vi "HAB Climber.vi"() -> ()   [LabVIEW 2018]
uses:
  <vilib>/Rock Robotics/SystemInterfaces/DIO/FPGA_DIOChannel.ctl
  <vilib>/Rock Robotics/WPI/ThirdParty/Phoenix-LabVIEW/Motor Controller/Controls/CTRE_Phoenix_MotorControl_ControlMode.ctl
  HAB Climber Global.vi
  <vilib>/Rock Robotics/WPI/Switch/WPI_SwitchOpenLimit.vi
  Times/Times Global.vi
  Controllers/Driver Controller/Driver Controller Global.vi
  Cargo Intake/Cargo Intake Global.vi
panel:
  out "HAB Lock":bool
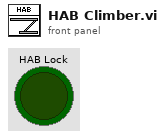
[diagram p1: front panel]
types:
  T1 = typedef "FPGA_DIOChannel.ctl" = enum8{"DIO 0", "DIO 1", "DIO 2", "DIO 3", "DIO 4", "DIO 5", "DIO 6", "DIO 7", "DIO 8", "DIO 9", "DIO MXP 0", "DIO MXP 1", "DIO MXP 2", "DIO MXP 3", "DIO MXP 4", "DIO MXP 5", "DIO MXP 6", "DIO MXP 7", "DIO MXP 8", "DIO MXP 9", "DIO MXP 10", "DIO MXP 11", "DIO MXP 12", "DIO MXP 13", "DIO MXP 14", "DIO MXP 15", "SPI Port CS1", "SPI Port CS2", "SPI Port CS3", "SPI Port MISO", "SPI Port MOSI", "Invalid"}
  T2 = enum16{"HAB Climber Full Manual Mode", "HAB Climber Manual Mode", "HAB Climber Automated Mode", "HAB Climber Fully Automated Mode"}
  T3 = typedef "WPI_SwitchDevRef.ctl" = cluster{"DevStatus":errorcluster, "DIO Channel":T1, "CntIndex":T4, "Normally Closed":bool}
  T4 = typedef "FPGA_CounterCtrSystemIndex.ctl" = enum8{"Ctr 0", "Ctr 1", "Ctr 2", "Ctr 3", "Ctr 4", "Ctr 5", "Ctr 6", "Ctr 7", "Invalid"}
  T5 = typedef "WPI_MotorControlDeviceRef.ctl" = cluster{"DeviceStatus":errorcluster, "Type":T6, "PWM":cluster{"PWM Channel":T7, "DeadBand":T8}, "CAN":cluster{"Device Number":u8, "SetOutput VI Ref":variant, "GetOutput VI Ref":variant, "Enable VI Ref":variant, "Disable VI Ref":variant, "Data":variant}, "Invert":bool, "DIO PWM":cluster{"PWM \"Enable\" Channel":T7, "DIOChannel":T1, "PWM Rate":dbl}}
  T6 = typedef "WPI_MotorControlType.ctl" = enum16{"PWM", "CAN", "DIO PWM"}
  T7 = typedef "FPGA_DIOPWMChannel.ctl" = enum8{"PWM 0", "PWM 1", "PWM 2", "PWM 3", "PWM 4", "PWM 5", "PWM 6", "PWM 7", "PWM 8", "PWM 9", "PWM MXP 0", "PWM MXP 1", "PWM MXP 2", "PWM MXP 3", "PWM MXP 4", "PWM MXP 5", "PWM MXP 6", "PWM MXP 7", "PWM MXP 8", "PWM MXP 9", "Invalid"}
  T8 = typedef "WPI_PWMDeadband.ctl" = cluster{"Name":string, "maxPositivePwm":i32, "minPositivePwm":i32, "centerPwm":i32, "maxNegativePwm":i32, "minNegativePwm":i32, "angularRange":u16}
  T9 = typedef "Control 3.ctl" = dbl
  T10 = typedef "CTRE_Phoenix_MotorControl_ControlMode.ctl" = u16
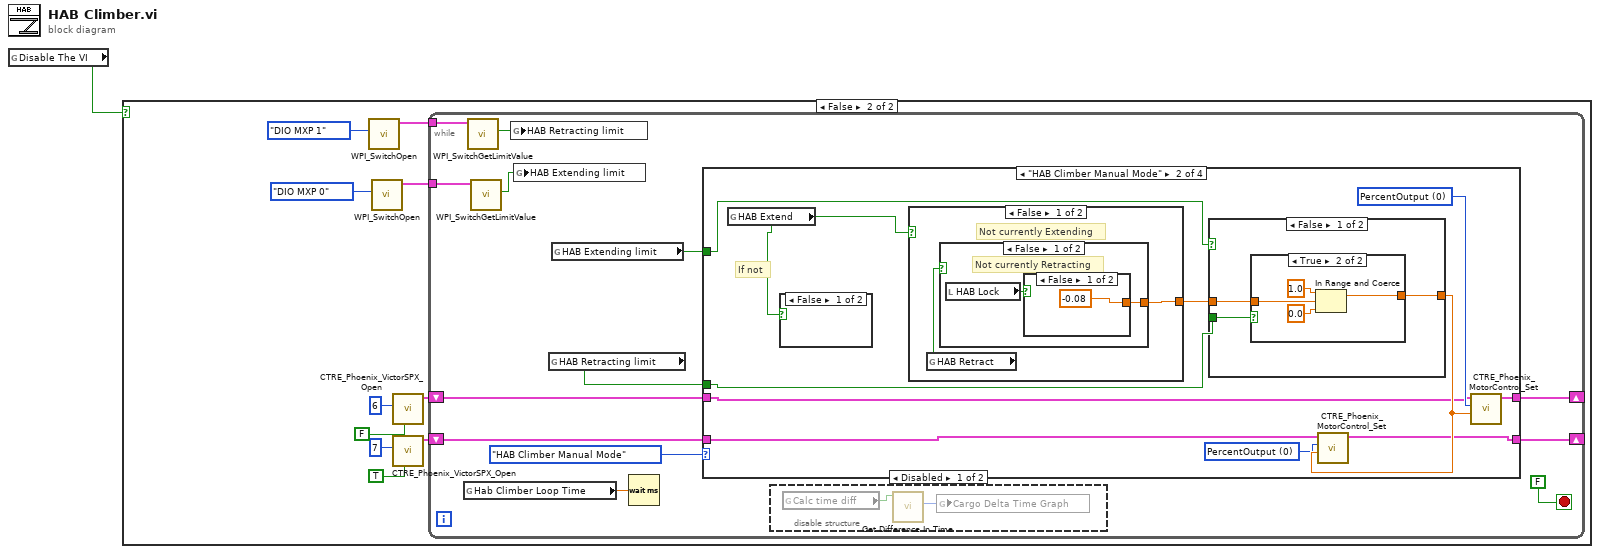
[diagram p0: block diagram]
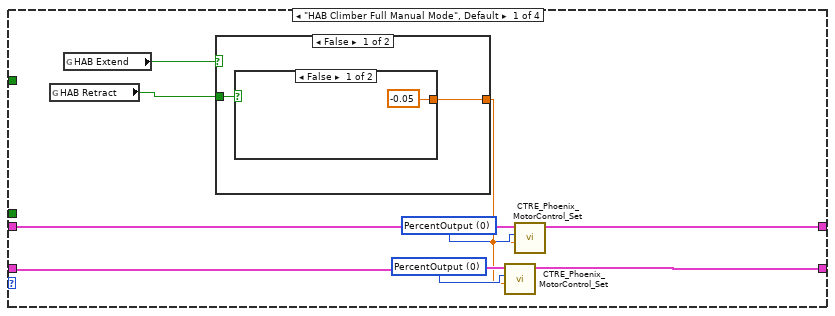
[diagram p4: hidden frame]
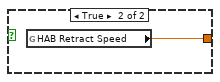
[diagram p5: hidden frame]
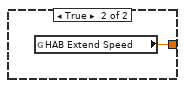
[diagram p6: hidden frame]
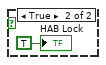
[diagram p7: hidden frame]
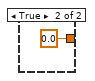
[diagram p8: hidden frame]
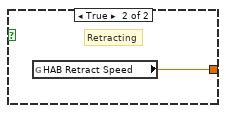
[diagram p9: hidden frame]
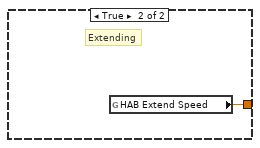
[diagram p10: hidden frame]
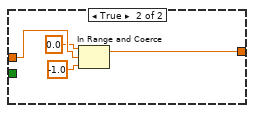
[diagram p12: hidden frame]
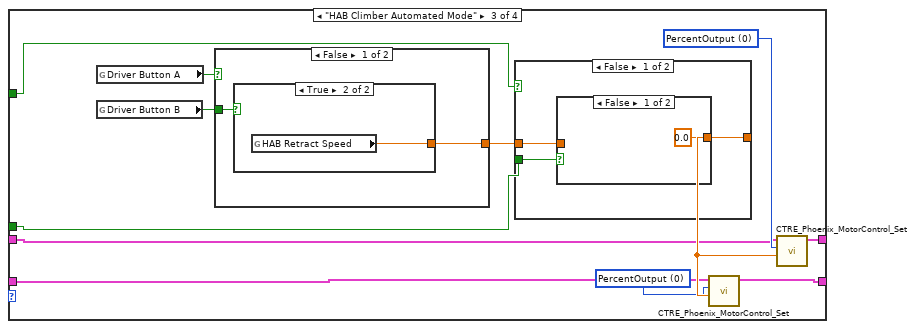
[diagram p13: hidden frame]
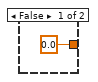
[diagram p14: hidden frame]
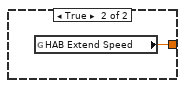
[diagram p15: hidden frame]
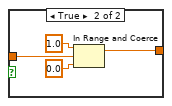
[diagram p16: hidden frame]
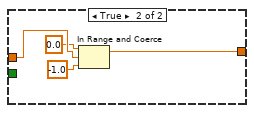
[diagram p17: hidden frame]
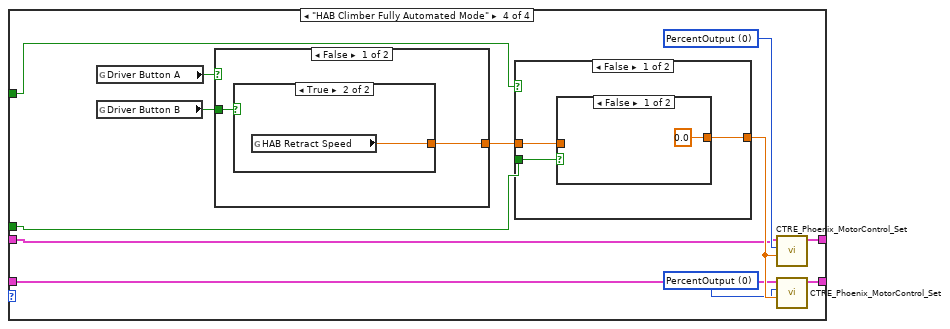
[diagram p18: hidden frame]
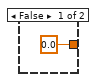
[diagram p19: hidden frame]
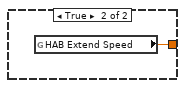
[diagram p20: hidden frame]
diagram:
  n1 = global read "HAB Climber Global.vi" "Disable The VI"() -> (w1:bool)
  n2 = case shown="False" w1 {
    frame True {
    }
    frame False {
      n3 = call-poly <vilib>:"WPI_SwitchOpen.vi"("DIO Channel"=FPGA_DIOChannel."DIO MXP 1") -> ("SwitchDevRef"=w5:T3)  [unwired: 9 in, 1 out]
      n4 = call-poly <vilib>:"WPI_SwitchOpen.vi"("DIO Channel"=FPGA_DIOChannel."DIO MXP 0") -> ("SwitchDevRef"=w4:T3)  [unwired: 9 in, 1 out]
      n5 = call <vilib>:"CTRE_Phoenix_VictorSPX_Open.vi"("Invert"=FALSE, "Device Number"=u8 6) -> ("CAN Talon SRX Ref"=w11:T5)  [unwired: 8 in, 1 out]
      n6 = call <vilib>:"CTRE_Phoenix_VictorSPX_Open.vi"("Invert"=TRUE, "Device Number"=u8 7) -> ("CAN Talon SRX Ref"=w9:T5)  [unwired: 8 in, 1 out]
      n7 = while {
        shift-right: [w19] -> _
        shift-left: w11 -> [w21]
        shift-right: [w18] -> _
        shift-left: w9 -> [w20]
        tunnel: w5 -> [w17]
        tunnel: w4 -> [w16]
        stop <- FALSE stop-if-true
        n8 = global read "Times Global.vi" "Hab Climber Loop Time"() -> (w24:T9)
        n9 = call <vilib>:"WPI_SwitchGetLimitValue.vi"("SwitchDevRef"=w17) -> ("Switch Pressed"=w12:bool)  [unwired: 8 in, 2 out]
        n10 = call <vilib>:"WPI_SwitchGetLimitValue.vi"("SwitchDevRef"=w16) -> ("Switch Pressed"=w13:bool)  [unwired: 8 in, 2 out]
        n11 = global write "HAB Climber Global.vi" "HAB Retracting limit"(w12) -> ()
        n12 = global write "HAB Climber Global.vi" "HAB Extending limit"(w13) -> ()
        n13 = global read "HAB Climber Global.vi" "HAB Retracting limit"() -> (w14:bool)
        n14 = global read "HAB Climber Global.vi" "HAB Extending limit"() -> (w15:bool)
        n15 = Wait (ms)(milliseconds to wait=w24) -> ()  [unwired: 1 out]
        n16 = case shown="\"HAB Climber Manual Mode\"" T2."HAB Climber Manual Mode" ("Mode") {
          tunnel: w21 -> [w32 w47 w78 w107]
          tunnel: w20 -> [w33 w46 w77 w106]
          tunnel: [w30 w45 w76 w105] -> w19
          tunnel: [w29 w44 w75 w104] -> w18
          tunnel: w15 -> [_ w43 w74 w103]
          tunnel: w14 -> [_ w42 w73 w102]
          frame "HAB Climber Full Manual Mode", Default {
            w34 = T10 0 items=["PercentOutput"=0, "Position"=1, "Velocity"=2, "Current"=3, "Follower"=5, "MotionProfile"=6, "MotionMagic"=7, "MotionProfileArc"=10, "Disabled"=15] ("Control Mode")
            w35 = T10 0 items=["PercentOutput"=0, "Position"=1, "Velocity"=2, "Current"=3, "Follower"=5, "MotionProfile"=6, "MotionMagic"=7, "MotionProfileArc"=10, "Disabled"=15] ("Control Mode")
            n17 = global read "HAB Climber Global.vi" "HAB Retract"() -> (w27:bool)
            n18 = global read "HAB Climber Global.vi" "HAB Extend"() -> (w28:bool)
            n19 = case shown="False" w28 {
              tunnel: w27 -> [w37 _]
              tunnel: [w36 w40] -> w31
              frame False {
                n20 = case shown="False" w37 {
                  tunnel: [-0.05 w39] -> w36
                  frame False {
                  }
                  frame True {
                    n21 = global read "HAB Climber Global.vi" "HAB Retract Speed"() -> (w39:dbl)
                  }
                }
              }
              frame True {
                n22 = global read "HAB Climber Global.vi" "HAB Extend Speed"() -> (w40:dbl)
              }
            }
            n23 = call <vilib>:"CTRE_Phoenix_MotorControl_Set.vi"("Output"=w31, "Control Mode"=w34, "PhoenixMotorControlDevRef"=w33) -> ("PhoenixMotorControlDevRef"=w29:T5)  [unwired: 7 in, 1 out]
            n24 = call <vilib>:"CTRE_Phoenix_MotorControl_Set.vi"("Output"=w31, "Control Mode"=w35, "PhoenixMotorControlDevRef"=w32) -> ("PhoenixMotorControlDevRef"=w30:T5)  [unwired: 7 in, 1 out]
          }
          frame "HAB Climber Manual Mode" {
            w48 = T10 0 items=["PercentOutput"=0, "Position"=1, "Velocity"=2, "Current"=3, "Follower"=5, "MotionProfile"=6, "MotionMagic"=7, "MotionProfileArc"=10, "Disabled"=15] ("Control Mode")
            w50 = T10 0 items=["PercentOutput"=0, "Position"=1, "Velocity"=2, "Current"=3, "Follower"=5, "MotionProfile"=6, "MotionMagic"=7, "MotionProfileArc"=10, "Disabled"=15] ("Control Mode")
            # "If not"
            n25 = global read "HAB Climber Global.vi" "HAB Extend"() -> (w41:bool)
            n26 = case shown="False" w41 {
              frame False {
              }
              frame True {
                "HAB Lock" <- TRUE ("HAB Lock")
              }
            }
            n27 = case shown="False" w41 {
              tunnel: [w54 w60] -> w51
              frame False {
                # "Not currently Extending"
                n28 = global read "HAB Climber Global.vi" "HAB Retract"() -> (w53:bool)
                n29 = case shown="False" w53 {
                  tunnel: [w56 w59] -> w54
                  frame False {
                    # "Not currently Retracting"
                    n30 = local read "HAB Lock"() -> (w55:bool)
                    n31 = case shown="False" w55 {
                      tunnel: [-0.08 0.0] -> w56
                      frame False {
                      }
                      frame True {
                      }
                    }
                  }
                  frame True {
                    # "Retracting"
                    n32 = global read "HAB Climber Global.vi" "HAB Retract Speed"() -> (w59:dbl)
                  }
                }
              }
              frame True {
                # "Extending"
                n33 = global read "HAB Climber Global.vi" "HAB Extend Speed"() -> (w60:dbl)
              }
            }
            n34 = case shown="False" w43 {
              tunnel: w51 -> [w62 w72]
              tunnel: [w63 w69] -> w49
              tunnel: w42 -> [w61 _]
              frame False {
                n35 = case shown="True" w61 {
                  tunnel: [w64 w68] -> w63
                  tunnel: w62 -> [w64 w67]
                  frame False {
                  }
                  frame True {
                    n36 = In Range and Coerce(upper limit=1.0, x=w67, lower limit=0.0) -> (coerced(x)=w68:dbl)  [unwired: 1 out]
                  }
                }
              }
              frame True {
                n37 = In Range and Coerce(upper limit=0.0, x=w72, lower limit=-1.0) -> (coerced(x)=w69:dbl)  [unwired: 1 out]
              }
            }
            n38 = call <vilib>:"CTRE_Phoenix_MotorControl_Set.vi"("Output"=w49, "Control Mode"=w48, "PhoenixMotorControlDevRef"=w46) -> ("PhoenixMotorControlDevRef"=w44:T5)  [unwired: 7 in, 1 out]
            n39 = call <vilib>:"CTRE_Phoenix_MotorControl_Set.vi"("Output"=w49, "Control Mode"=w50, "PhoenixMotorControlDevRef"=w47) -> ("PhoenixMotorControlDevRef"=w45:T5)  [unwired: 7 in, 1 out]
          }
          frame "HAB Climber Automated Mode" {
            w79 = T10 0 items=["PercentOutput"=0, "Position"=1, "Velocity"=2, "Current"=3, "Follower"=5, "MotionProfile"=6, "MotionMagic"=7, "MotionProfileArc"=10, "Disabled"=15] ("Control Mode")
            w80 = T10 0 items=["PercentOutput"=0, "Position"=1, "Velocity"=2, "Current"=3, "Follower"=5, "MotionProfile"=6, "MotionMagic"=7, "MotionProfileArc"=10, "Disabled"=15] ("Control Mode")
            n40 = global read "Driver Controller Global.vi" "Driver Button A"() -> (w82:bool)
            n41 = global read "Driver Controller Global.vi" "Driver Button B"() -> (w81:bool)
            n42 = case shown="False" w82 {
              tunnel: w81 -> [w86 _]
              tunnel: [w85 w89] -> w83
              frame False {
                n43 = case shown="True" w86 {
                  tunnel: [0.0 w88] -> w85
                  frame False {
                  }
                  frame True {
                    n44 = global read "HAB Climber Global.vi" "HAB Retract Speed"() -> (w88:dbl)
                  }
                }
              }
              frame True {
                n45 = global read "HAB Climber Global.vi" "HAB Extend Speed"() -> (w89:dbl)
              }
            }
            n46 = case shown="False" w74 {
              tunnel: w83 -> [w91 w101]
              tunnel: [w92 w98] -> w84
              tunnel: w73 -> [w90 _]
              frame False {
                n47 = case shown="False" w90 {
                  tunnel: [0.0 w97] -> w92
                  tunnel: w91 -> [_ w96]
                  frame False {
                  }
                  frame True {
                    n48 = In Range and Coerce(upper limit=1.0, x=w96, lower limit=0.0) -> (coerced(x)=w97:dbl)  [unwired: 1 out]
                  }
                }
              }
              frame True {
                n49 = In Range and Coerce(upper limit=0.0, x=w101, lower limit=-1.0) -> (coerced(x)=w98:dbl)  [unwired: 1 out]
              }
            }
            n50 = call <vilib>:"CTRE_Phoenix_MotorControl_Set.vi"("Output"=w84, "Control Mode"=w79, "PhoenixMotorControlDevRef"=w77) -> ("PhoenixMotorControlDevRef"=w75:T5)  [unwired: 7 in, 1 out]
            n51 = call <vilib>:"CTRE_Phoenix_MotorControl_Set.vi"("Output"=w84, "Control Mode"=w80, "PhoenixMotorControlDevRef"=w78) -> ("PhoenixMotorControlDevRef"=w76:T5)  [unwired: 7 in, 1 out]
          }
          frame "HAB Climber Fully Automated Mode" {
            w108 = T10 0 items=["PercentOutput"=0, "Position"=1, "Velocity"=2, "Current"=3, "Follower"=5, "MotionProfile"=6, "MotionMagic"=7, "MotionProfileArc"=10, "Disabled"=15] ("Control Mode")
            w109 = T10 0 items=["PercentOutput"=0, "Position"=1, "Velocity"=2, "Current"=3, "Follower"=5, "MotionProfile"=6, "MotionMagic"=7, "MotionProfileArc"=10, "Disabled"=15] ("Control Mode")
            n52 = global read "Driver Controller Global.vi" "Driver Button A"() -> (w111:bool)
            n53 = global read "Driver Controller Global.vi" "Driver Button B"() -> (w110:bool)
            n54 = case shown="False" w111 {
              tunnel: w110 -> [w115 _]
              tunnel: [w114 w118] -> w112
              frame False {
                n55 = case shown="True" w115 {
                  tunnel: [0.0 w117] -> w114
                  frame False {
                  }
                  frame True {
                    n56 = global read "HAB Climber Global.vi" "HAB Retract Speed"() -> (w117:dbl)
                  }
                }
              }
              frame True {
                n57 = global read "HAB Climber Global.vi" "HAB Extend Speed"() -> (w118:dbl)
              }
            }
            n58 = case shown="False" w103 {
              tunnel: w112 -> [w120 w130]
              tunnel: [w121 w127] -> w113
              tunnel: w102 -> [w119 _]
              frame False {
                n59 = case shown="False" w119 {
                  tunnel: [0.0 w126] -> w121
                  tunnel: w120 -> [_ w125]
                  frame False {
                  }
                  frame True {
                    n60 = In Range and Coerce(upper limit=1.0, x=w125, lower limit=0.0) -> (coerced(x)=w126:dbl)  [unwired: 1 out]
                  }
                }
              }
              frame True {
                n61 = In Range and Coerce(upper limit=0.0, x=w130, lower limit=-1.0) -> (coerced(x)=w127:dbl)  [unwired: 1 out]
              }
            }
            n62 = call <vilib>:"CTRE_Phoenix_MotorControl_Set.vi"("Output"=w113, "Control Mode"=w109, "PhoenixMotorControlDevRef"=w107) -> ("PhoenixMotorControlDevRef"=w105:T5)  [unwired: 7 in, 1 out]
            n63 = call <vilib>:"CTRE_Phoenix_MotorControl_Set.vi"("Output"=w113, "Control Mode"=w108, "PhoenixMotorControlDevRef"=w106) -> ("PhoenixMotorControlDevRef"=w104:T5)  [unwired: 7 in, 1 out]
          }
        }
        n64 = disable-structure shown="Disabled" {
          frame Disabled {
            n65 = global read "Cargo Intake Global.vi" "Calc time diff"() -> (w26:bool)
            n66 = call "Get Difference In Time.vi"("Calculate Time Difference"=w26) -> ("Delta Time over Time"=w25:u32)  [unwired: 9 in, 1 out]
            n67 = global write "Times Global.vi" "Cargo Delta Time Graph"(w25) -> ()
          }
          frame Enabled {
          }
        }
      }
    }
  }
